vi "AnimatorUninit.vi"(2 "Container State":T1, 3 "Display State":T2) -> ()   [LabVIEW 2013, in "AnimatorXControl.xctl"]
uses:
  AnimatorXControl.xctl
  AnimatorState.ctl
  <vilib>/picture/picture.llb/imagedata.ctl
  AnimatorSettings.ctl
  <vilib>/_xctls/Container State.ctl
  <vilib>/_xctls/XControlSupport.lvlib
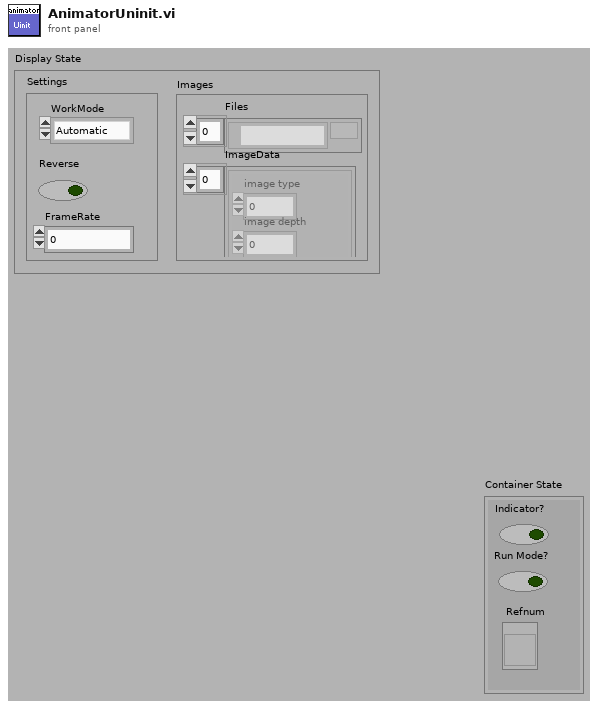
[diagram p1: front panel]
types:
  T1 = typedef "XControlSupport.lvlib/Container State.ctl" = cluster{"Indicator?":bool, "Run Mode?":bool, " Refnum":refnum<vi>}
  T2 = typedef "AnimatorXControl.xctl/AnimatorState.ctl" = cluster{"Images":cluster{"Files":path[], "ImageData":T3[]}, "Settings":T4}
  T3 = typedef "imagedata.ctl" = cluster{"image type":i32, "image depth":i32, "image":u8[], "mask":u8[], "colors":u32[], "Rectangle":cluster{"left":i16, "top":i16, "right":i16, "bottom":i16}}
  T4 = typedef "AnimatorXControl.xctl/AnimatorSettings.ctl" = cluster{"Reverse":bool, "FrameRate":dbl, "WorkMode":enum16{"Automatic", "UseValue"}}
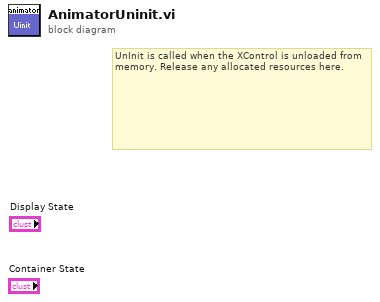
[diagram p0: block diagram]
diagram:
  # "UnInit is called when the XControl is unloaded from memory. Release any allocated resources here."
